vi "Alternate Start Async.vi"(7 "Queue of Self":refnum<queue>, 8 "Self Alias":string, 9 "Caller":refnum<data-value>, 10 "Caller Alias":string, 11 "Actor":refnum<class "Actor.lvclass">) -> (0 "error out":errorcluster)   [LabVIEW 2021, in "jettl Queue Actor.lvlib" / "jettl Queue Actor.lvclass"]
uses:
  jettl Queue Actor.lvclass
  Actor/Msg/Msg.lvclass
  Actor/Actor/Actor.lvclass
  Actor.vi
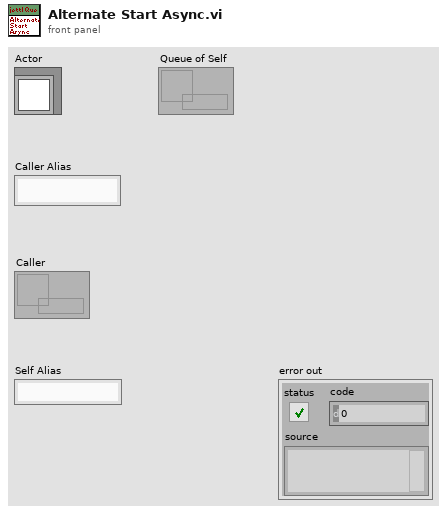
[diagram p1: front panel]
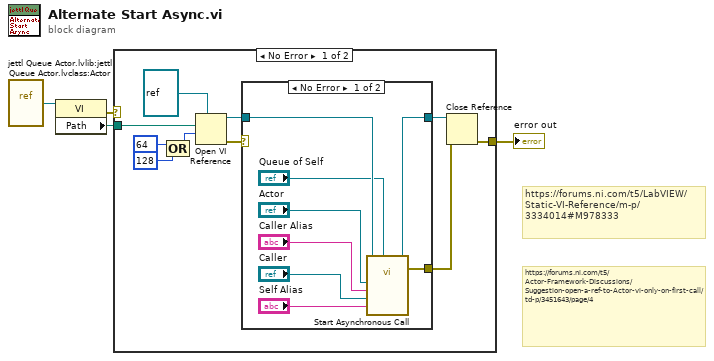
[diagram p0: block diagram]
diagram:
  # "https://forums.ni.com/t5/LabVIEW/Static-VI-Reference/m-p/3334014#M978333"
  # "https://forums.ni.com/t5/Actor-Framework-Discussions/Suggestion-open-a-ref-to-Actor-vi-only-on-first-call/td-p/3451643/page/4"
  n1 = vi-ref "jettl Queue Actor.lvlib:jettl Queue Actor.lvclass:Actor.vi"() -> (w3:refnum<vi>)
  n2 = property class="VI"(reference=w3) -> (error out=w4:errorcluster, "Path"=w2:path)  [unwired: 1 in, 1 out]
  n3 = case shown="No Error" w4 {
    selector: w4 -> [_ w25]
    tunnel: [w12 w25] -> w1
    tunnel: w2 -> [w8 _]
    frame No Error {
      n4 = Compound Arithmetic op=OR(64 ("options: Multiple Clones,\n  Fire & Forget"), 128 ("options: Multiple Clones,\n  Fire & Forget")) -> (w10:i32)
      n5 = Open VI Reference(type specifier VI Refnum (for type only)=refnum<vi> refnum, vi path=w8, options=w10) -> (vi reference=w6:refnum<vi>, error out=w7:errorcluster)  [unwired: 3 in]
      n6 = case shown="No Error" w7 {
        selector: w7 -> [_ w24]
        tunnel: [w22 w23] -> w14
        tunnel: [w21 w24] -> w13
        tunnel: w6 -> [w20 w23]
        frame No Error {
          n7 = call-by-ref "Start Asynchronous Call"(reference=w20, "Queue of Self"="Queue of Self", "Self Alias"="Self Alias", "Caller"="Caller", "Caller Alias"="Caller Alias", "Actor"="Actor") -> (reference out=w22:refnum<vi>, error out=w21:errorcluster)  [unwired: 8 in]
        }
        frame Error {
        }
      }
      n8 = Close Reference(reference=w14, error in (no error)=w13) -> (error out=w12:errorcluster)
    }
    frame Error {
    }
  }
  "error out" <- w1
